vi "Convert.BusDataArrayToStringArray.vi"(11 "frame":T1[](array[typedef])) -> (3 "Array out":string[][](array[string]))   [LabVIEW 2025, in "XNET Bus Monitor Client.lvlib"]
uses:
  XNET Bus Monitor Client.lvlib
  bus_monitor_client/RPC Messages/ni_bus_monitor_api_Frame.ctl
  <vilib>/Utility/error.llb/Trim Whitespace One-Sided.vi
  bus_monitor_client/bus_monitor_client.lvlib
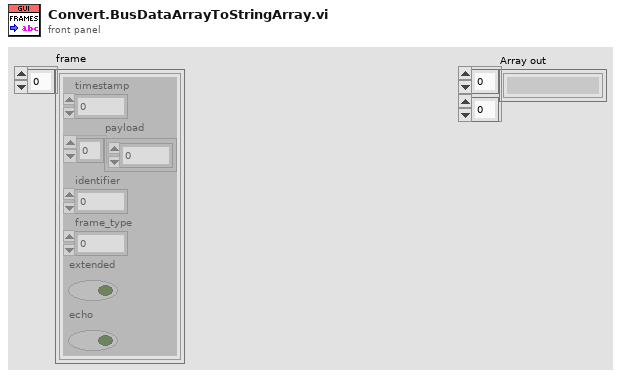
[diagram p1: front panel]
types:
  T1 = typedef "bus_monitor_client.lvlib/ni_bus_monitor_api_Frame.ctl" = cluster{"timestamp":dbl, "payload":u8[], "identifier":u32, "frame_type":u32, "extended":bool, "echo":bool}
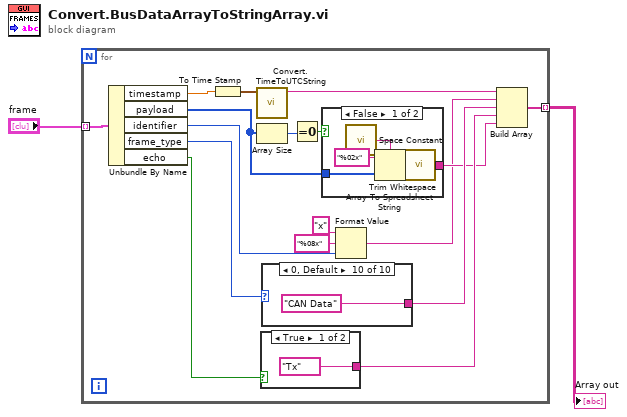
[diagram p0: block diagram]
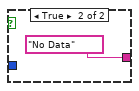
[diagram p2: hidden frame]
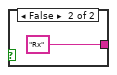
[diagram p3: hidden frame]
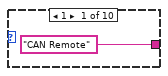
[diagram p4: hidden frame]
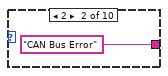
[diagram p5: hidden frame]
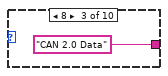
[diagram p6: hidden frame]
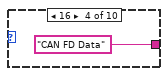
[diagram p7: hidden frame]
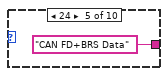
[diagram p8: hidden frame]
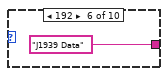
[diagram p9: hidden frame]
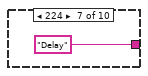
[diagram p10: hidden frame]
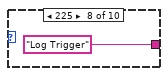
[diagram p11: hidden frame]
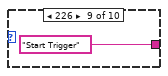
[diagram p12: hidden frame]
diagram:
  n1 = for {
    tunnel: "frame" -> [w19] mode=indexing
    tunnel: [w7] -> w1 mode=indexing
    n2 = Unbundle By Name(w19) -> ("timestamp"=w18:dbl, "payload"=w11:u8[], "identifier"=w17:u32, "frame_type"=w16:u32, "echo"=w14:bool)
    n3 = To Time Stamp(1:w18) -> (0:w3:timestamp)
    n4 = call "Convert.TimeToUTCString.vi"("timestamp"=w3) -> ("UTC string"=w9:string)  [unwired: 10 in]
    n5 = Array Size(array=w11) -> (size(s)=w13:i32)
    n6 = case shown="True" w14 {
      tunnel: ["Tx" "Rx"] -> w10
      frame True {
      }
      frame False {
      }
    }
    n7 = case shown="0, Default" w16 {
      tunnel: ["CAN Remote" "CAN Bus Error" "CAN 2.0 Data" "CAN FD Data" "CAN FD+BRS Data" "J1939 Data" "Delay" "Log Trigger" "Start Trigger" "CAN Data"] -> w15
      frame 1 {
      }
      frame 2 {
      }
      frame 8 {
      }
      frame 16 {
      }
      frame 24 {
      }
      frame 192 {
      }
      frame 224 {
      }
      frame 225 {
      }
      frame 226 {
      }
      frame 0, Default {
      }
    }
    n8 = Equal To 0?(x=w13) -> (x = 0?=w12:bool)
    n9 = case shown="False" w12 {
      tunnel: [w20 "No Data"] -> w8
      tunnel: w11 -> [w24 _]
      frame False {
        n10 = call <vilib>:"Space Constant.vi"() -> ("String"=w21:string)
        n11 = Array To Spreadsheet String(delimiter (Tab)=w21, array=w24, 3:"%02x" ("format string")) -> (spreadsheet string=w23:string)
        n12 = call <vilib>:"Trim Whitespace.vi"("string"=w23) -> ("trimmed string"=w20:string)  [unwired: 1 in]
      }
      frame True {
      }
    }
    n13 = Format Value(string ("")="x" ("string"), format string="%08x", value (0)=w17) -> (output string=w4:string)
    n14 = Build Array(w9, w4, w15, w10, w8) -> (w7:string[])
  }
  "Array out" <- w1
